vi "createModel.vi"(8 "error in (no error)":errorcluster, 11 "Boot in":refnum<class "Boot.lvclass">) -> (0 "error out":errorcluster, 2 "Model":refnum<class "Model.lvclass">, 3 "Boot out":refnum<class "Boot.lvclass">)   [LabVIEW 2016, in "Boot.lvclass"]
uses:
  Boot.lvclass
  Model/Model.lvclass
  Model/Model.lvclass/Model.ctl
  Boot.lvclass/Boot.ctl
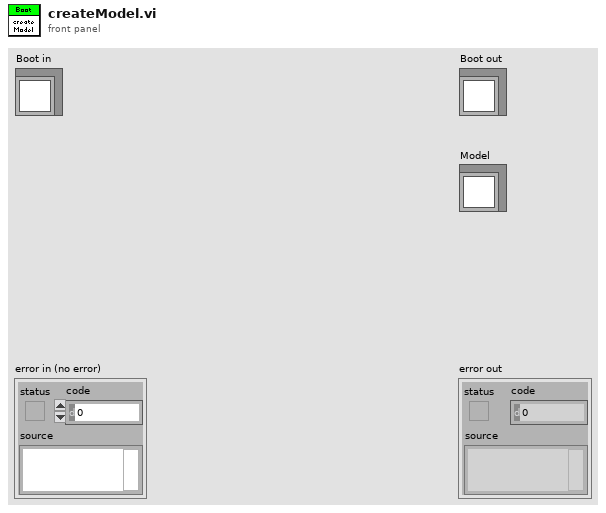
[diagram p1: front panel]
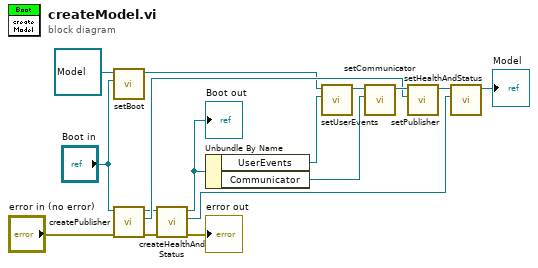
[diagram p0: block diagram]
diagram:
  n1 = call "setBoot.vi"("Boot"="Boot in", "Model in"=refnum<class "Model.lvclass"> refnum ("Model.lvclass")) -> ("Model out"=w1:refnum<class "Model.lvclass">)  [unwired: 9 in]
  n2 = call "createPublisher.vi"("error in (no error)"="error in (no error)", "Boot in"="Boot in") -> ("error out"=w5:errorcluster, "Publisher"=w10:refnum<class "Publisher.lvclass">, "Boot out"=w9:refnum<class "Boot.lvclass">)  [unwired: 7 in]
  n3 = call "createHealthAndStatus.vi"("error in (no error)"=w5, "Boot in"=w9) -> ("error out"=→"error out":errorcluster, "HealthAndStatus"=w8:refnum<class "RTHealthAndStatus.lvclass">, "Boot out"=w7:refnum<class "Boot.lvclass">)  [unwired: 7 in]
  "Boot out" <- w7
  n4 = Unbundle By Name(w7) -> ("UserEvents"=w15:refnum<class "UserEvents.lvclass">, "Communicator"=w14:refnum<class "Communicator.lvclass">)
  n5 = call "setUserEvents.vi"("UserEvents"=w15, "Model in"=w1) -> ("Model out"=w16:refnum<class "Model.lvclass">)  [unwired: 9 in]
  n6 = call "setCommunicator.vi"("Communicator"=w14, "Model in"=w16) -> ("Model out"=w13:refnum<class "Model.lvclass">)  [unwired: 9 in]
  n7 = call "setPublisher.vi"("Publisher"=w10, "Model in"=w13) -> ("Model out"=w12:refnum<class "Model.lvclass">)  [unwired: 9 in]
  n8 = call "setHealthAndStatus.vi"("HealthAndStatus"=w8, "Model in"=w12) -> ("Model out"=→"Model":refnum<class "Model.lvclass">)  [unwired: 9 in]
